vi "P6.vi"() -> ()   [LabVIEW 2019]
uses:
  <vilib>/Utility/file.llb/Write Delimited Spreadsheet (DBL).vi
panel:
  in  "operation (0:open)":T1(ring)
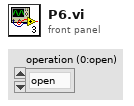
[diagram p1: front panel]
types:
  T1 = enum16{"open", "replace", "create", "open or create", "replace or create", "replace or create with confirmation"}
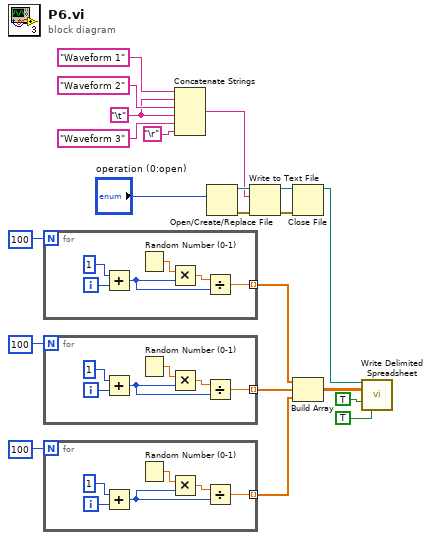
[diagram p0: block diagram]
diagram:
  w13 = "\t"
  n1 = for {
    N: 100 -> [_]
    tunnel: [w22] -> w7 mode=indexing
    i -> [w27]
    n2 = Add(x=1, y=w27) -> (x+y=w23:i32)
    n3 = Random Number (0-1)() -> (number: 0 to 1=w25:dbl)
    n4 = Multiply(x=w25, y=w23) -> (x*y=w24:dbl)
    n5 = Divide(x=w24, y=w23) -> (x/y=w22:dbl)
  }
  n6 = for {
    N: 100 -> [_]
    tunnel: [w28] -> w8 mode=indexing
    i -> [w33]
    n7 = Add(x=1, y=w33) -> (x+y=w29:i32)
    n8 = Random Number (0-1)() -> (number: 0 to 1=w31:dbl)
    n9 = Multiply(x=w31, y=w29) -> (x*y=w30:dbl)
    n10 = Divide(x=w30, y=w29) -> (x/y=w28:dbl)
  }
  n11 = for {
    N: 100 -> [_]
    tunnel: [w34] -> w9 mode=indexing
    i -> [w39]
    n12 = Add(x=1, y=w39) -> (x+y=w35:i32)
    n13 = Random Number (0-1)() -> (number: 0 to 1=w37:dbl)
    n14 = Multiply(x=w37, y=w35) -> (x*y=w36:dbl)
    n15 = Divide(x=w36, y=w35) -> (x/y=w34:dbl)
  }
  n16 = Concatenate Strings("Waveform 1", w13, "Waveform 2", w13, "Waveform 3", "\r") -> (w16:string)
  n17 = Open/Create/Replace File(operation (0:open)="operation (0:open)") -> (refnum out=w20:refnum<file>, error out=w18:errorcluster)  [unwired: 5 in, 1 out]
  n18 = Write to Text File(file (use dialog)=w20, text=w16, error in=w18) -> (refnum out=w19:refnum<file>, error out=w17:errorcluster)  [unwired: 1 in, 1 out]
  n19 = Close File(refnum=w19, error in=w17) -> (path=w6:path)  [unwired: 1 out]
  n20 = Build Array(w7, w8, w9) -> (w10:dbl[][])
  n21 = call-poly <vilib>:"Write Delimited Spreadsheet.vi"("file path (dialog if empty)"=w6, "2D data"=w10, "append to file? (new file:F)"=TRUE, "transpose? (no:F)"=TRUE) -> ()  [unwired: 10 in, 2 out]
